vi "lab2_test.vi"() -> ()   [LabVIEW 2019]
uses:
  <vilib>/Platform/TimedLoop/XDataNode/timing_clust.ctl
  <vilib>/Platform/TimedLoop/XDataNode/nitl_modes.ctl
  <vilib>/Platform/TimedLoop/XDataNode/wakeup.ctl
  <vilib>/Analysis/3filter.llb/Filter Passband Type.ctl
  <vilib>/DAQmx/read.llb/DAQmx Read (Analog DBL 1Chan 1Samp).vi
  <vilib>/DAQmx/create/channels.llb/DAQmx Create Channel (AI-Voltage-Basic).vi
  <vilib>/DAQmx/miscellaneous.llb/DAQmx Fill In Error Info.vi
  <vilib>/platform/TimedLoop/XDataNode/XDataNode.xnode
  <vilib>/Platform/TimedLoop/XDataNode/XDNodeRunTimeDep.lvlib
  <vilib>/Analysis/NI_AALBase.lvlib
  <vilib>/ptbypt/NI_PtbyPt.lvlib
panel:
  out "Raw Position":dbl
  out "Raw Position Graph":dbl(graph)
  out "Raw Acceleration":dbl
  out "Raw Velocity":dbl
  out "Filtered Velocity":dbl
  out "Filtered Velocity Graph":dbl(graph)
  in  "low cutoff freq:  Velocity":dbl=0.125 format="%0.3f"
  out "Filtered Acceleration":dbl
  out "Filtered Acceleration Graph":dbl(graph)
  in  "low cutoff freq: Acceleration":dbl=0.125 format="%0.3f"
  out "Raw Acceleration Graph":dbl(graph)
  out "Raw Veloctiy Graph":dbl(graph)
  in  "low cutoff freq: Position":dbl=0.125 format="%0.3f"
  out "Filtered Postion Graph":dbl(graph)
  out "Filtered Position":dbl
  in  "STOP":bool
  out "Position":dbl(knob) scale=-32.5..32.5
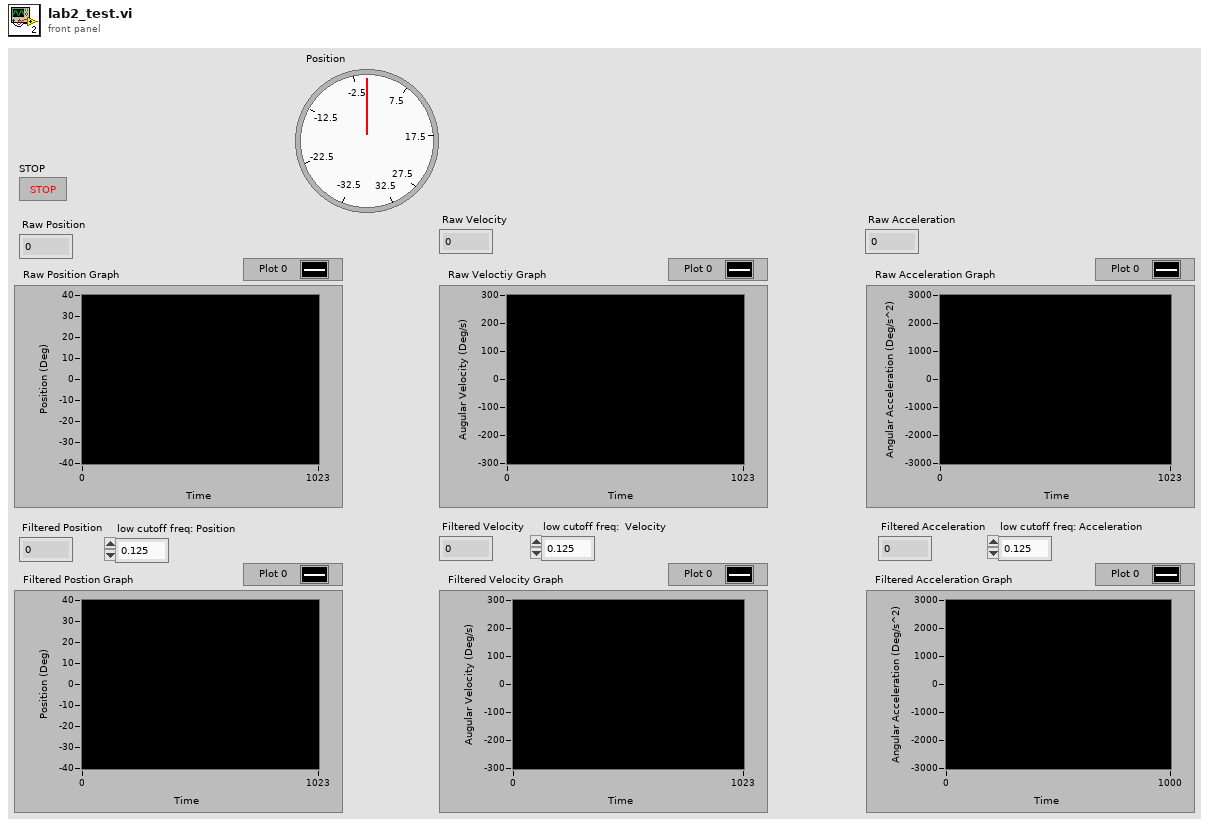
[diagram p1: front panel]
types:
  T1 = typedef "NI_AALBase.lvlib/Filter Passband Type.ctl" = enum32{"Lowpass", "Highpass", "Bandpass", "Bandstop"}
  T2 = typedef "XDNodeRunTimeDep.lvlib/timing_clust.ctl" = cluster{"Expected End [f-1]":u64, "Actual End [f-1]":u64, "Finished Late? [f-1]":bool, "Expected End [i-1]":u64, "Actual End [i-1]":u64, "Finished Late? [i-1]":bool, "Expected Start [i]":u64, "Actual Start [i]":u64, "Expected Start [f]":u64, "Actual Start [f]":u64, "Source Name":string, "Structure Name":string, "Period":i64, "Deadline":i64, "Offset":i64, "Start":i64, "Priority":i32, "Timeout":i32, "Mode":T3, "Wakeup Reason":T4, "Error":errorcluster, "Source Type":string, "Secondary Source Type":string, "Global End Time":u64, "Global Start Time":u64, "Frame Duration":u64, "Iteration Duration":u64, "Assigned CPU":i32, "I/O Scan Engine Mode":u32}
  T3 = typedef "XDNodeRunTimeDep.lvlib/nitl_modes.ctl" = enum32{"No Change", "Process missed periods, maintain original phase", "Discard missed periods, maintain original phase", "Process missed periods, ignore original phase", "Discard missed periods, ignore original phase"}
  T4 = typedef "XDNodeRunTimeDep.lvlib/wakeup.ctl" = enum32{"Normal", "Aborted", "Asynchronous wakeup", "Timing source error", "Timed loop error", "Timeout"}
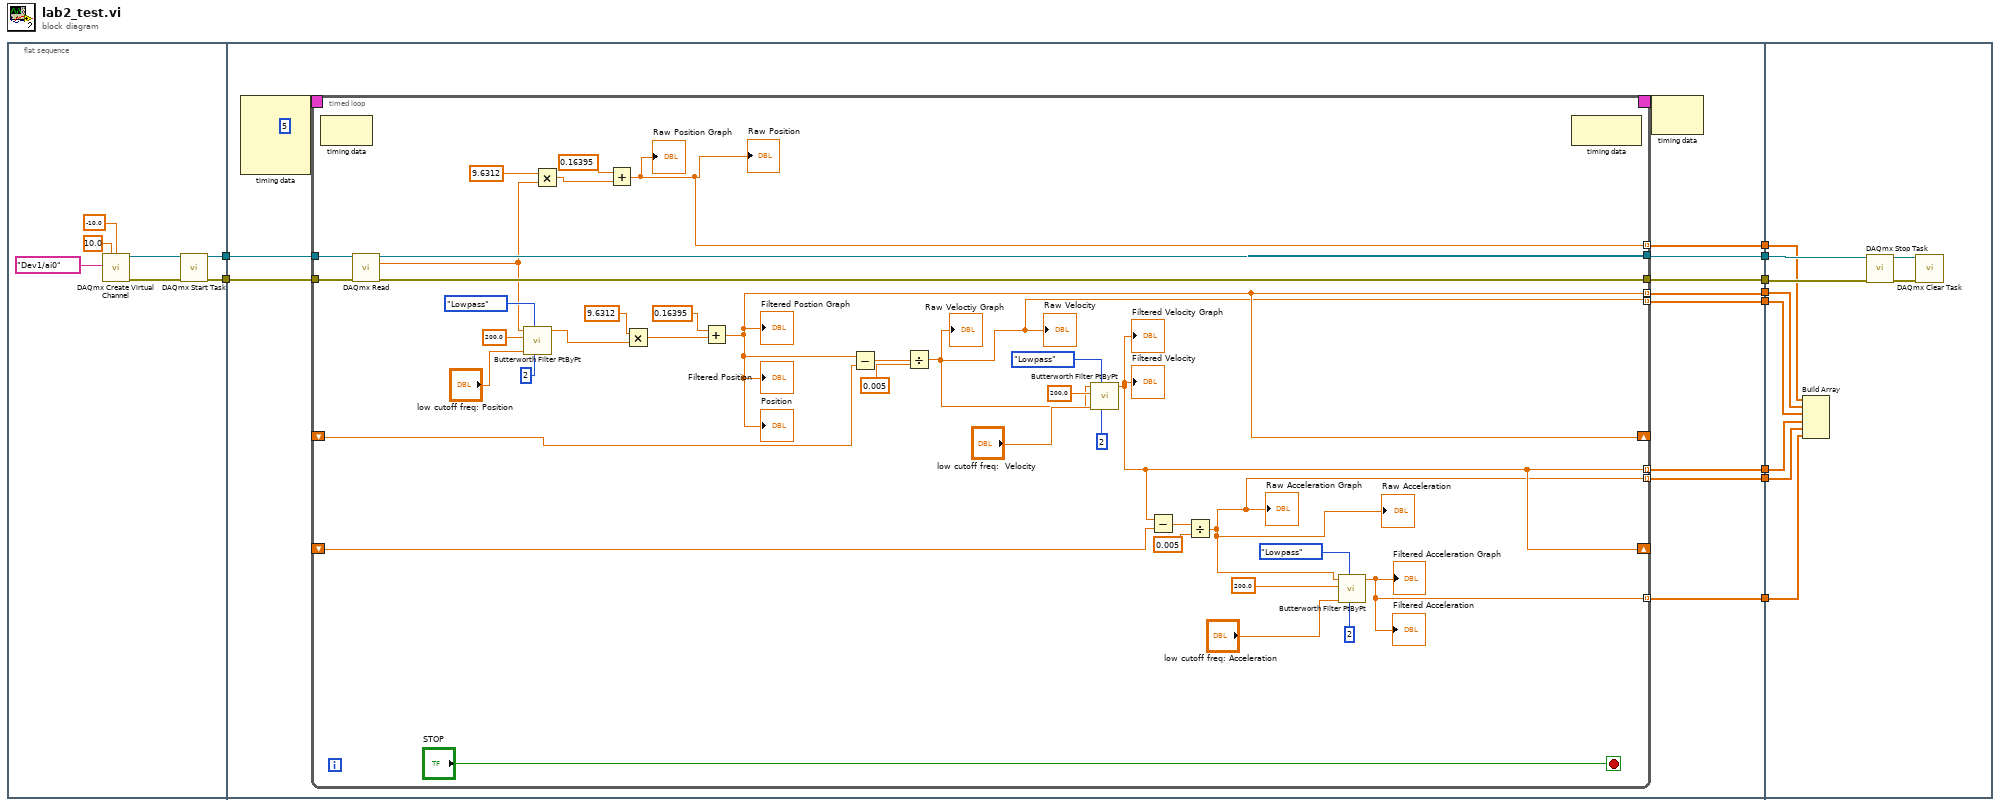
[diagram p0: block diagram]
diagram:
  n1 = flat-sequence {
    tunnel: [w13] -> w10
    tunnel: [w11] -> w9
    tunnel: w10 -> [w28]
    tunnel: [w27] -> w8
    tunnel: w9 -> [w26]
    tunnel: [w24] -> w7
    tunnel: [w23] -> w6
    tunnel: [w22] -> w5
    tunnel: [w21] -> w4
    tunnel: [w20] -> w3
    tunnel: [w19] -> w2
    tunnel: [w18] -> w1
    tunnel: w8 -> [w83]
    tunnel: w7 -> [w81]
    tunnel: w6 -> [w78]
    tunnel: w5 -> [w76]
    tunnel: w4 -> [w74]
    tunnel: w3 -> [w79]
    tunnel: w2 -> [w77]
    tunnel: w1 -> [w75]
    frame #0 {
      n2 = call-poly <vilib>:"DAQmx Create Virtual Channel.vi"("maximum value"=10.0, "minimum value"=-10.0, "physical channels"=tag "Dev1/ai0") -> ("task out"=w12:refnum<k21>, "error out"=w14:errorcluster)  [unwired: 11 in]
      n3 = call <vilib>:"DAQmx Start Task.vi"("task/channels in"=w12, "error in"=w14) -> ("task out"=w11:refnum<k21>, "error out"=w13:errorcluster)  [unwired: 12 in]
    }
    frame #1 {
      n4 = node-c288(i64 5 ("Period")) -> (w30:T2)  [unwired: 3 in]
      n5 = timed-loop {
        timing: w30 -> [_]
        timing-out: [_] -> w29
        tunnel: w28 -> [w67]
        tunnel: [w66] -> w27
        tunnel: w26 -> [w61]
        tunnel: [w60] -> w24
        shift-right: [w37] -> _
        shift-left: _ -> [w38]
        shift-right: [w36] -> _
        shift-left: _ -> [w57]
        tunnel: [w37] -> w23 mode=indexing
        tunnel: [w36] -> w22 mode=indexing
        tunnel: [w35] -> w21 mode=indexing
        tunnel: [w34] -> w20 mode=indexing
        tunnel: [w33] -> w19 mode=indexing
        tunnel: [w32] -> w18 mode=indexing
        stop <- "STOP" stop-if-true
        n6 = node-c288() -> ()  [unwired: 1 in, 1 out]
        n7 = call-poly <vilib>:"DAQmx Read.vi"("task/channels in"=w61, "error in"=w67) -> ("task out"=w60:refnum<k21>, "data"=w43:dbl, "error out"=w66:errorcluster)  [unwired: 11 in]
        n8 = call <vilib>:"Butterworth Filter PtByPt.vi"("order"=2, "filter type"=Filter_Passband_Type."Lowpass", "low cutoff freq: fl"="low cutoff freq: Position", "sampling freq: fs"=200.0, "x"=w43) -> ("Filtered x"=w39:dbl)  [unwired: 4 in, 1 out]
        n9 = Multiply(x=9.6312, y=w43) -> (x*y=w45:dbl)
        n10 = Add(x=0.16395, y=w45) -> (x+y=w34:dbl)
        "Raw Position Graph" <- w34
        "Raw Position" <- w34
        n11 = Multiply(x=9.6312, y=w39) -> (x*y=w41:dbl)
        n12 = Add(x=0.16395, y=w41) -> (x+y=w37:dbl)
        "Filtered Postion Graph" <- w37
        "Filtered Position" <- w37
        "Position" <- w37
        n13 = Subtract(x=w37, y=w38) -> (x-y=w59:dbl)
        n14 = Divide(x=w59, y=0.005) -> (x/y=w33:dbl)
        "Raw Veloctiy Graph" <- w33
        "Raw Velocity" <- w33
        n15 = call <vilib>:"Butterworth Filter PtByPt.vi"("order"=2, "filter type"=Filter_Passband_Type."Lowpass", "low cutoff freq: fl"="low cutoff freq:  Velocity", "sampling freq: fs"=200.0, "x"=w33) -> ("Filtered x"=w36:dbl)  [unwired: 4 in, 1 out]
        "Filtered Velocity Graph" <- w36
        "Filtered Velocity" <- w36
        n16 = Subtract(x=w36, y=w57) -> (x-y=w56:dbl)
        n17 = Divide(x=w56, y=0.005) -> (x/y=w32:dbl)
        "Raw Acceleration Graph" <- w32
        "Raw Acceleration" <- w32
        n18 = call <vilib>:"Butterworth Filter PtByPt.vi"("order"=2, "filter type"=Filter_Passband_Type."Lowpass", "low cutoff freq: fl"="low cutoff freq: Acceleration", "sampling freq: fs"=200.0, "x"=w32) -> ("Filtered x"=w35:dbl)  [unwired: 4 in, 1 out]
        "Filtered Acceleration Graph" <- w35
        "Filtered Acceleration" <- w35
        n19 = node-c288() -> ()  [unwired: 1 in, 1 out]
      }
      n20 = node-c288(w29) -> ()  [unwired: 1 out]
    }
    frame #2 {
      n21 = Build Array(w79, w78, w77, w76, w75, w74) -> ()  [unwired: 1 out]
      n22 = call <vilib>:"DAQmx Stop Task.vi"("task/channels in"=w81, "error in"=w83) -> ("task out"=w80:refnum<k21>, "error out"=w82:errorcluster)  [unwired: 12 in]
      n23 = call <vilib>:"DAQmx Clear Task.vi"("task in"=w80, "error in"=w82) -> ()  [unwired: 13 in, 1 out]
    }
  }
